vi "Read ADU Packet.vi"(8 "error in":errorcluster, 10 "isMaster (f)":bool, 11 "RTU transmission data unit in":refnum<class "RTU Data Unit.lvclass">) -> (0 "error out":errorcluster, 1 "modbus data unit":refnum<class "Modbus Data Unit.lvclass">, 3 "RTU transmission data unit out":refnum<class "RTU Data Unit.lvclass">, 5 "PDU Valid?":bool)   [LabVIEW 2021, in "RTU Data Unit.lvclass"]
doc: "This uses the protocol layer to read a modbus packet off of the bus, wrapped in the RTU transmission data unit."
uses:
  RTU Data Unit.lvclass
  D:/my_projects/projects/Algorithms/Labview/21/Modbus_v121c/Transmission Data Unit/Transmission Data Unit.lvclass
  D:/my_projects/projects/Algorithms/Labview/21/Modbus_v121c/Transmission Data Unit/Serial Interface/Serial Data Unit.lvclass
  Modbus Data Unit/Modbus Data Unit.lvclass
  Network Interface/Serial Interface/Serial Interface.lvclass
  D:/my_projects/projects/Algorithms/Labview/21/Modbus_v121c/Network Interface/Network Interface.lvclass
  Transmission Data Unit.lvclass/Transmission Data Unit.ctl
  Network Interface/Serial Interface/Serial Interface.lvclass/Serial Interface.ctl
  RTU Data Unit.lvclass/RTU Data Unit.ctl
  Serial Interface/Serial Data Unit.lvclass/Serial Data Unit.ctl
  Modbus Data Unit/Modbus Data Unit.lvclass/Modbus Data Unit.ctl
  Serial Interface/Serial acquisition states.ctl
  buffer element.ctl
  <vilib>/ErrorRing/Error Ring.xnode
  Network Interface/Network Interface.lvclass
  Serial Interface/Serial Data Unit.lvclass
  Transmission Data Unit.lvclass
  Network Protocol/Serial Shared Components/Serial Shared Components.lvlib
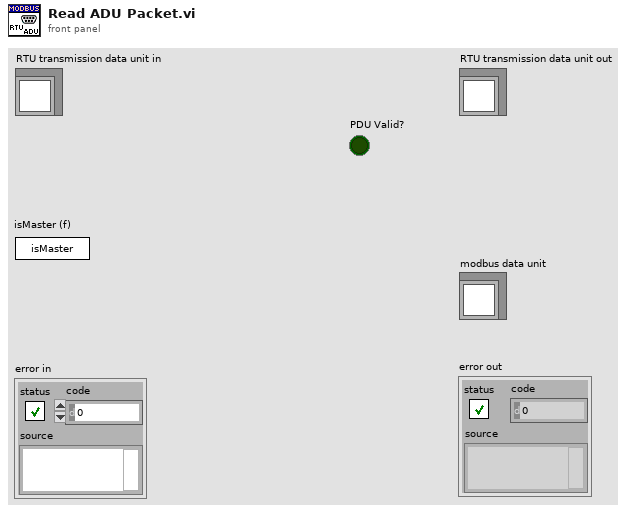
[diagram p1: front panel]
types:
  T1 = typedef "RTU Data Unit.lvclass/buffer element.ctl" = cluster{"data":u8[], "packets contained":i32}
  T2 = typedef "Serial Data Unit.lvclass/Serial acquisition states.ctl" = enum16{"Wait for frame", "Check for validity"}
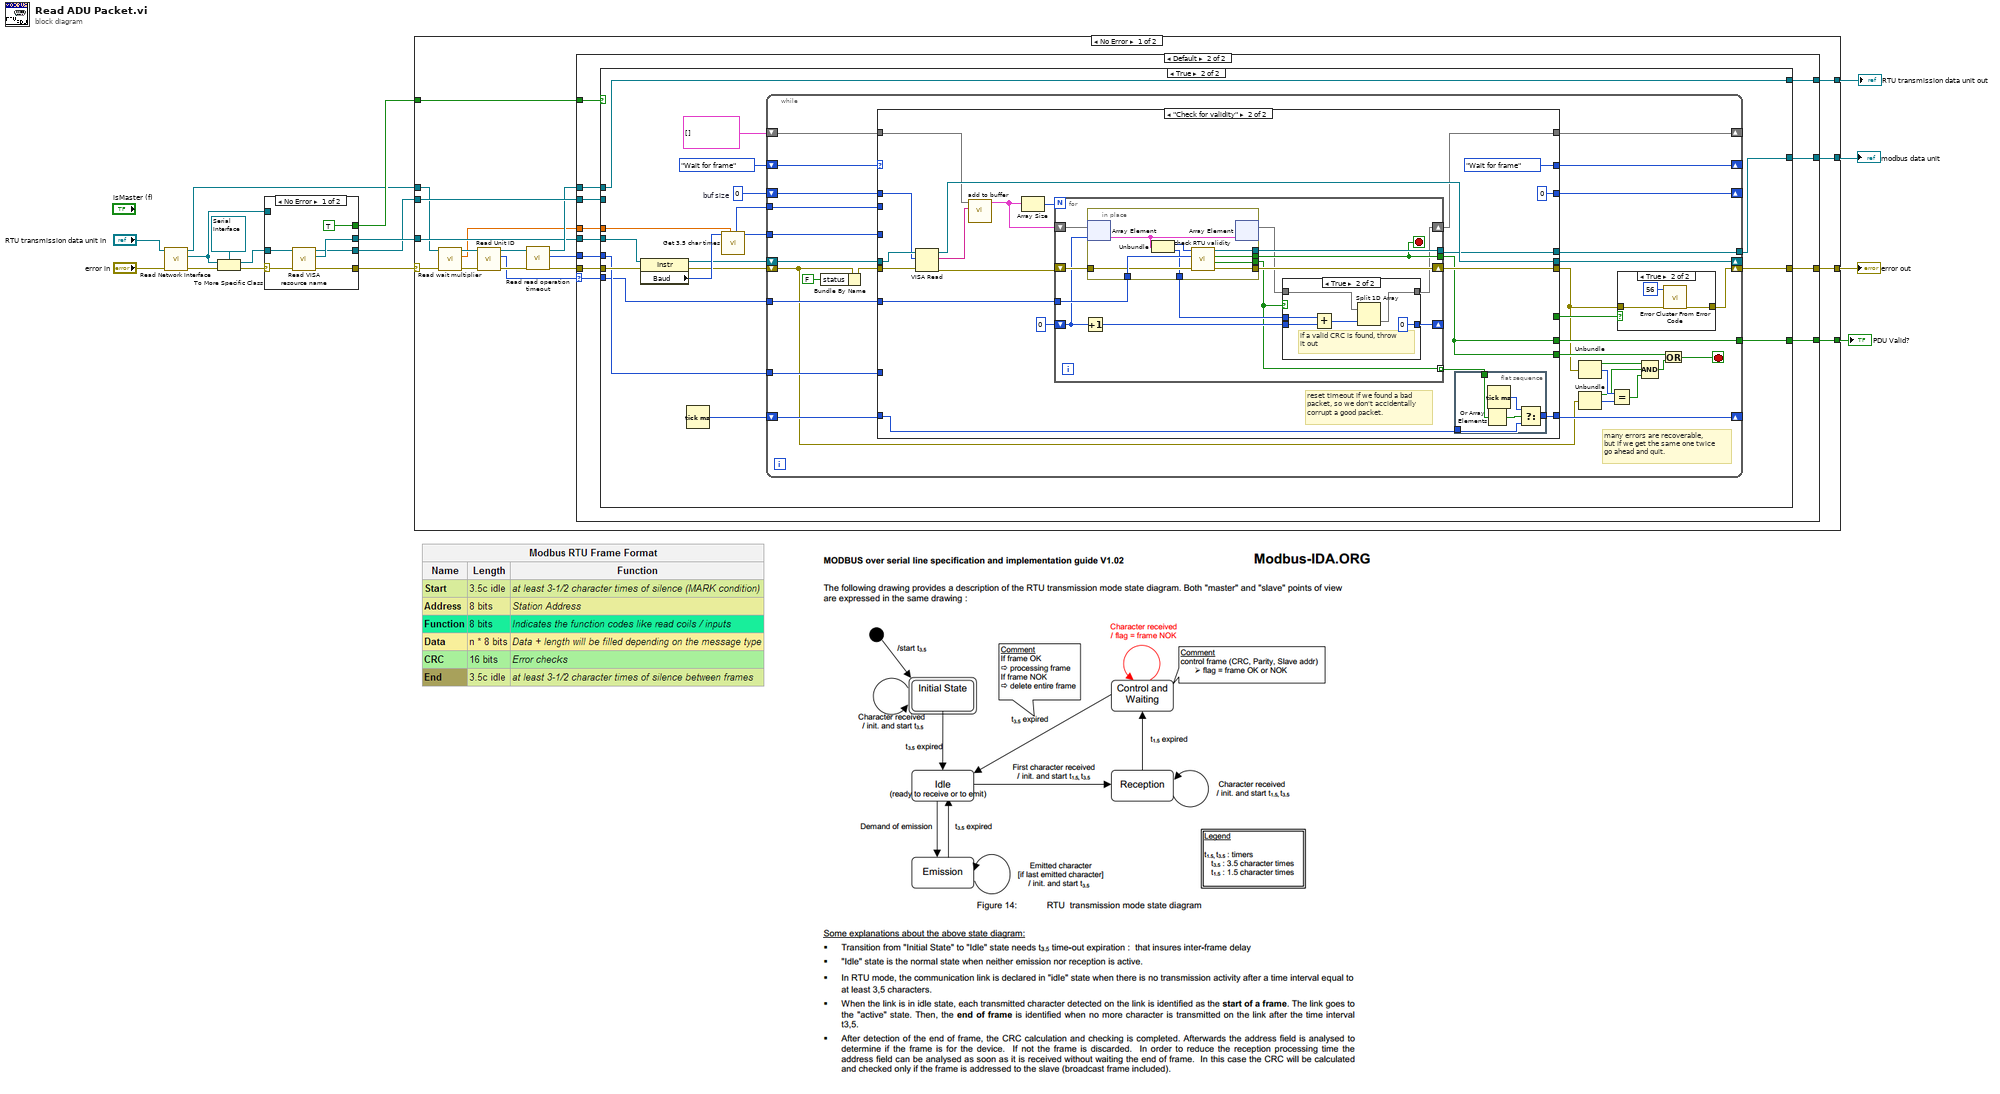
[diagram p0: block diagram]
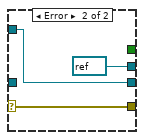
[diagram p2: hidden frame]
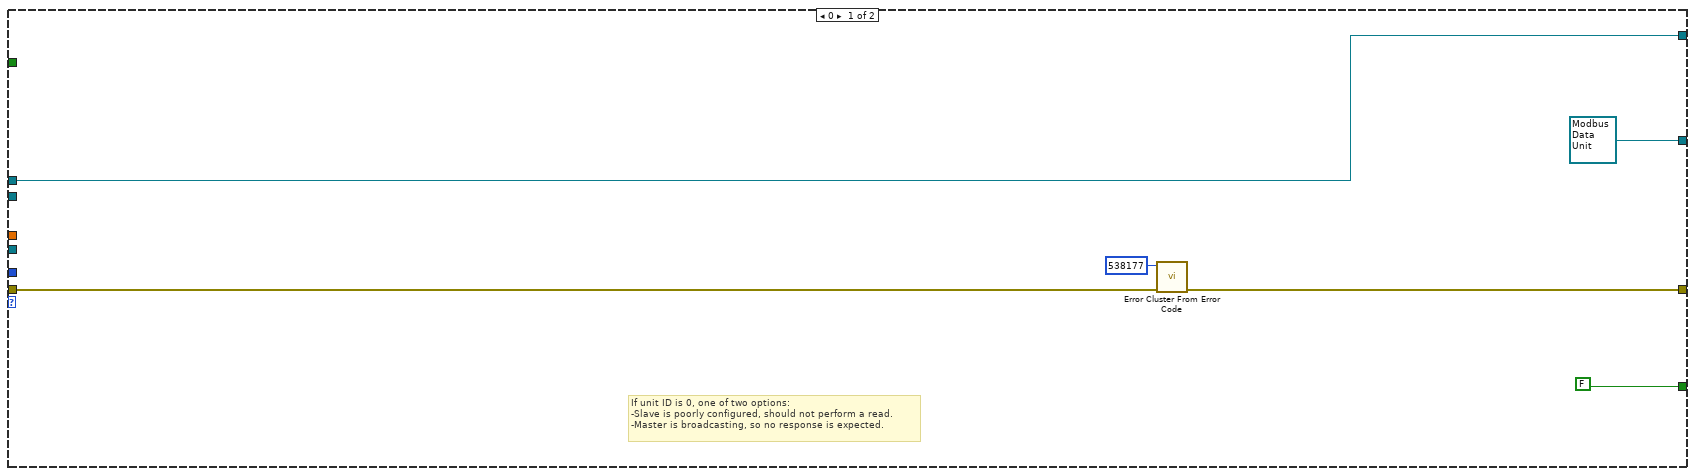
[diagram p3: hidden frame]
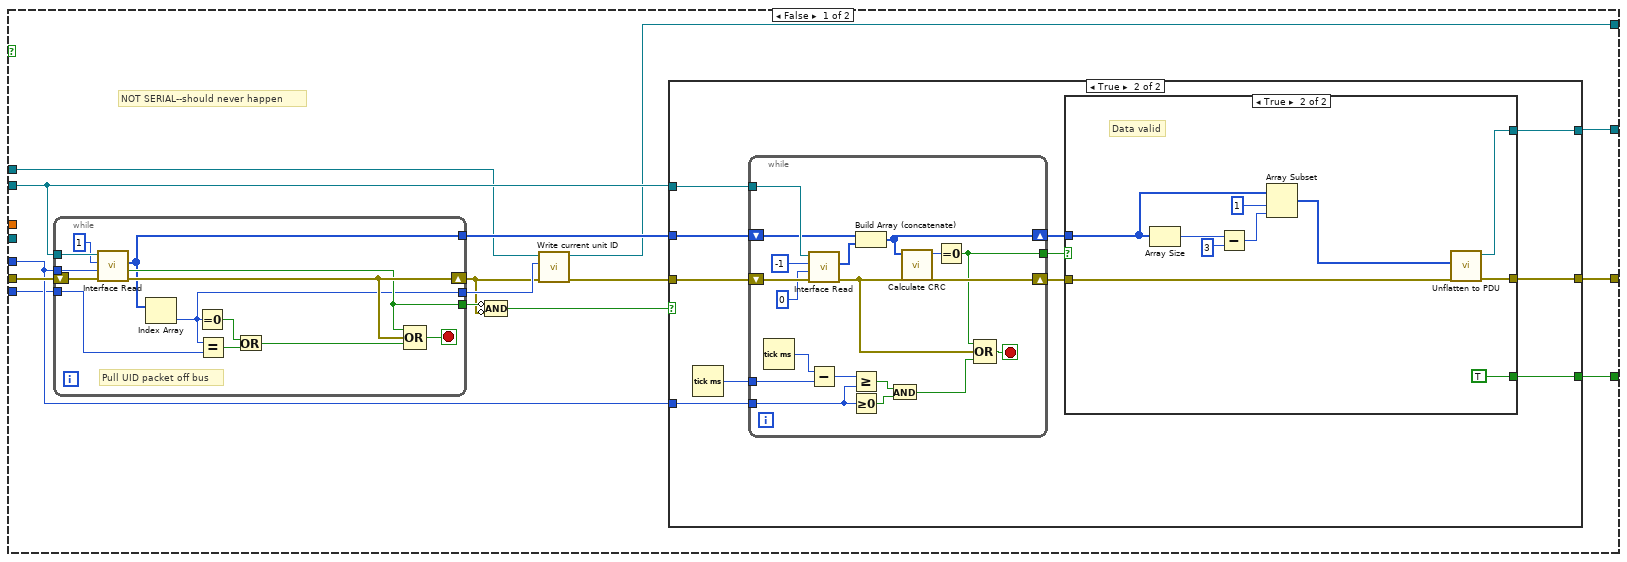
[diagram p4: hidden frame]
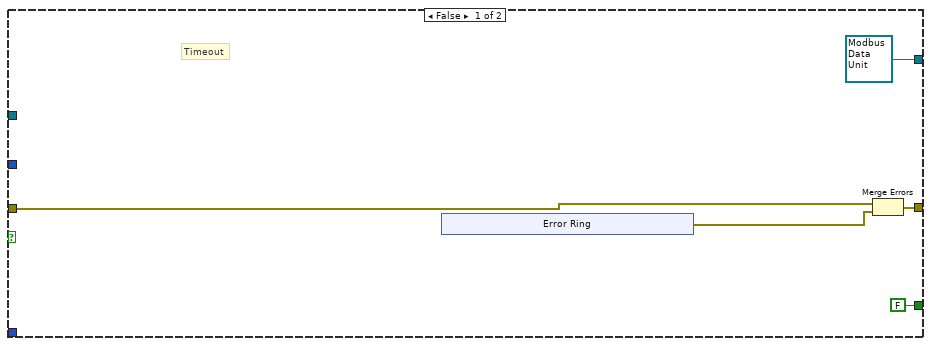
[diagram p5: hidden frame]
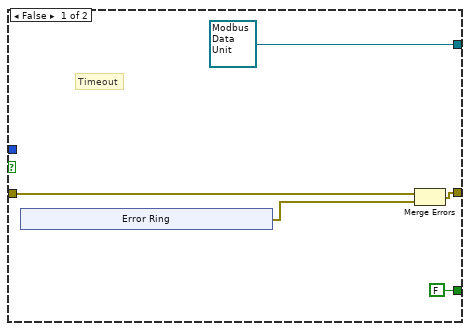
[diagram p6: hidden frame]
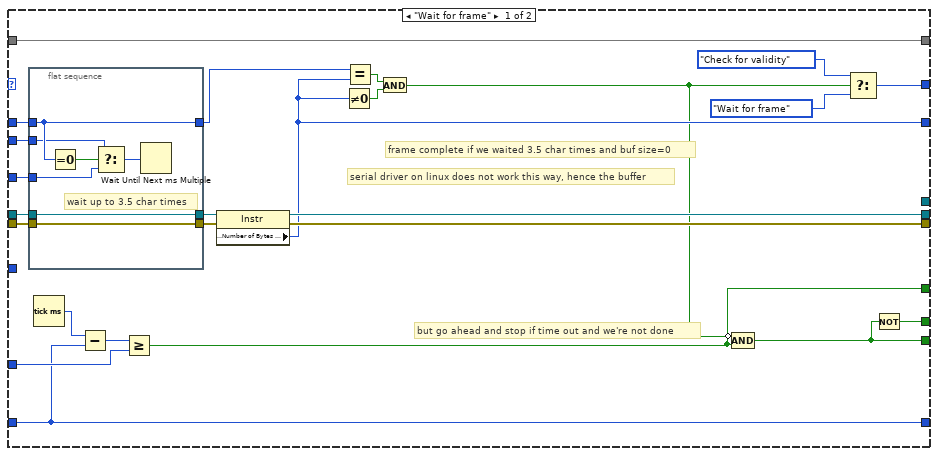
[diagram p8: hidden frame]
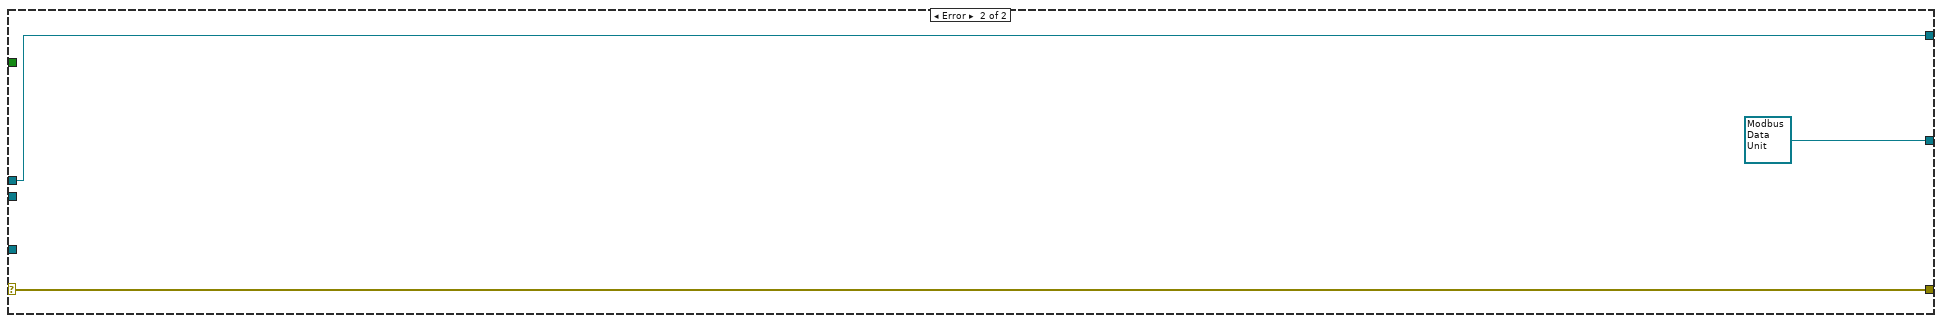
[diagram p10: hidden frame]
diagram:
  n1 = call "Read Network Interface.vi"("error in (no error)"="error in", "Transmission Data Unit in"="RTU transmission data unit in") -> ("error out"=w5:errorcluster, "Network Interface"=w4:refnum<class "Network Interface.lvclass">, "Transmission Data Unit out"=w3:refnum<class "RTU Data Unit.lvclass">)  [unwired: 7 in]
  n2 = To More Specific Class(target class=refnum<class "Serial Interface.lvclass"> refnum ("Serial Interface"), reference=w4, error in=w5) -> (specific class reference=w15:refnum<class "Serial Interface.lvclass">, error out=w16:errorcluster)
  n3 = case shown="No Error" w16 {
    selector: w16 -> [w21 w25]
    tunnel: [TRUE _] -> w13
    tunnel: [w19 refnum<visa-resource-name> refnum ("VISA resource name")] -> w14
    tunnel: w15 -> [w20 _]
    tunnel: [w18 w24] -> w1
    tunnel: [w17 w25] -> w2
    tunnel: w4 -> [_ w24]
    frame No Error {
      n4 = call "Read VISA resource name.vi"("error in (no error)"=w21, "Serial Master in"=w20) -> ("error out"=w17:errorcluster, "VISA resource name"=w19:refnum<visa-resource-name>, "Serial Master out"=w18:refnum<class "Serial Interface.lvclass">)  [unwired: 7 in]
    }
    frame Error {
    }
  }
  n5 = case shown="No Error" w2 {
    selector: w2 -> [w29 w288]
    tunnel: [w43 w288] -> w10
    tunnel: w3 -> [w30 w286]
    tunnel: w1 -> [w41 _]
    tunnel: [w42 refnum<class "Modbus Data Unit.lvclass"> refnum ("modbus data unit")] -> w11
    tunnel: [w40 w286] -> w12
    tunnel: [w33 _] -> w9
    tunnel: w13 -> [w32 _]
    tunnel: w14 -> [w31 _]
    frame No Error {
      n6 = call "Read wait multiplier.vi"("error in (no error)"=w29, "RTU Data Unit in"=w30) -> ("error out"=w28:errorcluster, "wait multiplier"=w26:sgl, "RTU Data Unit out"=w27:refnum<class "RTU Data Unit.lvclass">)  [unwired: 7 in]
      n7 = call "Read Unit ID.vi"("error in"=w28, "transmission data unit in"=w27) -> ("error out"=w37:errorcluster, "unit ID"=w35:u8, "transmission data unit out"=w36:refnum<class "RTU Data Unit.lvclass">)  [unwired: 7 in]
      n8 = call "Read read operation timeout.vi"("error in (no error)"=w37, "transmission data unit in"=w36) -> ("error out"=w38:errorcluster, "read operation timeout"=w34:i32, "transmission data unit out"=w39:refnum<class "RTU Data Unit.lvclass">)  [unwired: 7 in]
      n9 = case shown="Default" w35 {
        selector: w35 -> [_ w56]
        tunnel: w38 -> [w49 w61]
        tunnel: [w45 w60] -> w43
        tunnel: [refnum<class "Modbus Data Unit.lvclass"> refnum ("modbus data unit out") w59] -> w42
        tunnel: w41 -> [_ w58]
        tunnel: w34 -> [_ w57]
        tunnel: w39 -> [w48 w54]
        tunnel: [w48 w55] -> w40
        tunnel: [FALSE w53] -> w33
        tunnel: w32 -> [_ w52]
        tunnel: w31 -> [_ w51]
        tunnel: w26 -> [_ w50]
        frame 0 {
          # "If unit ID is 0, one of two options:\n-Slave is poorly configured, should not perform a read.\n-Master is broadcasting, so no response is expected."
          n10 = call <vilib>:"Error Cluster From Error Code.vi"("error in (no error)"=w49, "error code (0)"=538177) -> ("error out"=w45:errorcluster)  [unwired: 7 in]
        }
        frame Default {
          n11 = case shown="True" w52 {
            tunnel: w61 -> [w76 w162]
            tunnel: [w73 w159] -> w60
            tunnel: [w72 w150] -> w59
            tunnel: w58 -> [w71 _]
            tunnel: w57 -> [w69 w154]
            tunnel: w56 -> [w68 w151]
            tunnel: [w67 w164] -> w55
            tunnel: w54 -> [w65 w164]
            tunnel: [w62 w152] -> w53
            tunnel: w51 -> [_ w161]
            tunnel: w50 -> [_ w147]
            frame False {
              # "NOT SERIAL--should never happen"
              n12 = while {
                shift-right: [w143] -> w63
                shift-left: w76 -> [w146]
                tunnel: w69 -> [w141]
                tunnel: w68 -> [w137]
                tunnel: [w136] -> w75
                tunnel: [w135] -> w70
                tunnel: w71 -> [w145]
                tunnel: [w134] -> w64
                stop <- w144 stop-if-true
                # "Pull UID packet off bus"
                n13 = call-dynamic "Interface Read.vi"("error in"=w146, "timeout"=w141, "bytes to read"=1, "interface in"=w145) -> ("error out"=w143:errorcluster, "timed out?"=w136:bool, "data"=w135:u8[])  [unwired: 4 in, 1 out]
                n14 = Index Array(array=w135) -> (element=w134:u8)  [unwired: 1 in]
                n15 = Equal To 0?(x=w134) -> (x = 0?=w138:bool)
                n16 = Equal?(x=w134, y=w137) -> (x = y?=w140:bool)
                n17 = Or(x=w138, y=w140) -> (x .or. y?=w139:bool)
                n18 = Compound Arithmetic op=OR(w136, w143, w139) -> (w144:bool)
              }
              n19 = Compound Arithmetic op=AND(invert w75, invert w63) -> (w74:bool)
              n20 = call "Write current unit ID.vi"("error in"=w63, "request unit ID"=w64, "Serial Data Unit in"=w65) -> ("error out"=w66:errorcluster, "Serial Data Unit out"=w67:refnum<class "RTU Data Unit.lvclass">)  [unwired: 7 in]
              n21 = case shown="True" w74 {
                tunnel: w66 -> [w79 w96]
                tunnel: [w80 w88] -> w73
                tunnel: [refnum<class "Modbus Data Unit.lvclass"> refnum ("modbus data unit out") w89] -> w72
                tunnel: w71 -> [_ w92]
                tunnel: w70 -> [_ w93]
                tunnel: w69 -> [_ w94]
                tunnel: [FALSE w86] -> w62
                frame False {
                  # "Timeout"
                  n22 = xnode "Error Ring"() -> ("error out"=w81:errorcluster)
                  n23 = Merge Errors(w79, w81) -> (w80:errorcluster)
                }
                frame True {
                  n24 = Tick Count (ms)() -> (millisecond timer value=w95:u32)
                  n25 = while {
                    shift-right: [w119] -> w90
                    shift-left: w96 -> [w125]
                    tunnel: w95 -> [w133]
                    tunnel: w94 -> [w130]
                    shift-right: [w117] -> w87
                    shift-left: w93 -> [w121]
                    tunnel: w92 -> [w124]
                    tunnel: [w116] -> w91
                    stop <- w127 stop-if-true
                    n26 = Tick Count (ms)() -> (millisecond timer value=w132:u32)
                    n27 = call-dynamic "Interface Read.vi"("error in"=w125, "timeout"=0, "bytes to read"=-1, "interface in"=w124) -> ("error out"=w119:errorcluster, "data"=w120:u8[])  [unwired: 4 in, 2 out]
                    n28 = Subtract(x=w132, y=w133) -> (x-y=w131:u32)
                    n29 = Greater Or Equal?(x=w131, y=w130) -> (x >= y?=w128:bool)
                    n30 = Greater Or Equal To 0?(x=w130) -> (x >= 0?=w129:bool)
                    n31 = Build Array (concatenate)(w121, w120) -> (w117:u8[])
                    n32 = And(x=w128, y=w129) -> (x .and. y?=w126:bool)
                    n33 = call "Calculate CRC.vi"("data"=w117) -> ("CRC-16"=w118:u16)  [unwired: 10 in]
                    n34 = Equal To 0?(x=w118) -> (x = 0?=w116:bool)
                    n35 = Compound Arithmetic op=OR(w116, w119, w126) -> (w127:bool)
                  }
                  n36 = case shown="True" w91 {
                    tunnel: w90 -> [w99 w113]
                    tunnel: [refnum<class "Modbus Data Unit.lvclass"> refnum ("modbus data unit") w114] -> w89
                    tunnel: [w98 w115] -> w88
                    tunnel: w87 -> [_ w107]
                    tunnel: [FALSE TRUE] -> w86
                    frame False {
                      # "Timeout"
                      n37 = xnode "Error Ring"() -> ("error out"=w100:errorcluster)
                      n38 = Merge Errors(w99, w100) -> (w98:errorcluster)
                    }
                    frame True {
                      # "Data valid"
                      n39 = Array Size(array=w107) -> (size(s)=w111:i32)
                      n40 = Subtract(x=w111, y=3) -> (x-y=w109:i32)
                      n41 = Array Subset(array=w107, index=1, length=w109) -> (w108:u8[])
                      n42 = call "Unflatten to PDU.vi"("error in"=w113, "modbus data unit data"=w108) -> ("error out"=w115:errorcluster, "modbus data unit out"=w114:refnum<class "Modbus Data Unit.lvclass">)  [unwired: 8 in]
                    }
                  }
                }
              }
            }
            frame True {
              w156 = u32 0  # buf size
              n43 = property class="Instr"(reference=w161, error in=w162) -> (reference out=w158:refnum<visa-resource-name>, error out=w160:errorcluster, "Baud"=w163:u32)
              n44 = Tick Count (ms)() -> (millisecond timer value=w155:u32)
              n45 = call "Get 3.5 char times.vi"("wait multiplier"=w147, "baud rate"=w163) -> ("wait time (ms)"=w153:u32, "initial wait (ms)"=w149:u32)  [unwired: 8 in]
              n46 = while {
                shift-right: [w181] -> w159
                shift-left: w160 -> [w171]
                shift-right: [w187] -> _
                shift-left: w158 -> [w193]
                shift-right: [w186] -> _
                shift-left: Serial_acquisition_states."Wait for frame" ("Serial Acquisition States") -> [w194]
                shift-right: [w188] -> _
                shift-left: w156 -> [w190]
                tunnel: w154 -> [w191]
                tunnel: w153 -> [w189]
                tunnel: [w185] -> w152
                tunnel: w151 -> [w184]
                tunnel: [w183] -> w150
                tunnel: w149 -> [w180]
                shift-right: [w178] -> _
                shift-left: T1[] [] -> [w179]
                shift-right: [w177] -> _
                shift-left: w155 -> [w192]
                stop <- w174 stop-if-true
                # "many errors are recoverable,\nbut if we get the same one twice\ngo ahead and quit."
                n47 = Bundle By Name(cluster=w171, "status"=FALSE) -> (w176:errorcluster)
                n48 = case shown="\"Check for validity\"" w194 {
                  tunnel: w193 -> [w219 w249]
                  tunnel: w176 -> [w218 w250]
                  tunnel: w192 -> [w199 w232]
                  tunnel: w191 -> [w221 _]
                  tunnel: w190 -> [w216 w248]
                  tunnel: w189 -> [w215 _]
                  tunnel: [w206 u32 0 ("Bytes at Port")] -> w188
                  tunnel: [w203 w233] -> w173
                  tunnel: [w211 w243] -> w172
                  tunnel: [w210 w242] -> w187
                  tunnel: [w207 Serial_acquisition_states."Wait for frame" ("Serial Acquisition States")] -> w186
                  tunnel: [w204 w233] -> w185
                  tunnel: w184 -> [_ w246]
                  tunnel: [_ w240] -> w183
                  tunnel: [w202 _] -> w182
                  tunnel: w180 -> [w201 _]
                  tunnel: w179 -> [w200 w239]
                  tunnel: [w200 w235] -> w178
                  tunnel: [w199 w234] -> w177
                  frame "Wait for frame" {
                    # "serial driver on linux does not work this way, hence the buffer"
                    # "but go ahead and stop if time out and we're not done"
                    # "frame complete if we waited 3.5 char times and buf size=0"
                    n49 = flat-sequence {
                      tunnel: [w230] -> w220
                      tunnel: w219 -> [w230]
                      tunnel: w218 -> [w229]
                      tunnel: [w229] -> w217
                      tunnel: w216 -> [w228]
                      tunnel: [w228] -> w212
                      tunnel: w215 -> [w226]
                      tunnel: w201 -> [w224]
                      frame #0 {
                        # "wait up to 3.5 char times"
                        n50 = Equal To 0?(x=w228) -> (x = 0?=w227:bool)
                        n51 = Select(t=w224, s=w227, f=w226) -> (s? t:f=w225:u32)
                        n52 = Wait Until Next ms Multiple(millisecond multiple=w225) -> ()  [unwired: 1 out]
                      }
                    }
                    n53 = Tick Count (ms)() -> (millisecond timer value=w223:u32)
                    n54 = Subtract(x=w223, y=w199) -> (x-y=w222:u32)
                    n55 = Greater Or Equal?(x=w222, y=w221) -> (x >= y?=w202:bool)
                    n56 = property class="Instr"(reference=w220, error in=w217) -> (reference out=w210:refnum<visa-resource-name>, error out=w211:errorcluster, "Serial Settings:Number of Bytes at Serial Port"=w206:u32)
                    n57 = Not Equal To 0?(x=w206) -> (x != 0?=w214:bool)
                    n58 = Equal?(x=w212, y=w206) -> (x = y?=w213:bool)
                    n59 = And(x=w213, y=w214) -> (x .and. y?=w205:bool)
                    n60 = Compound Arithmetic op=AND(invert w205, w202) -> (w203:bool)
                    n61 = Select(t=Serial_acquisition_states."Check for validity" ("Serial Acquisition States"), s=w205, f=Serial_acquisition_states."Wait for frame" ("Serial Acquisition States")) -> (s? t:f=w207:T2)
                    n62 = Not(x=w203) -> (.not. x?=w204:bool)
                  }
                  frame "Check for validity" {
                    # "reset timeout if we found a bad\npacket, so we don't accidentally\ncorrupt a good packet."
                    n63 = VISA Read(VISA resource name=w249, byte count=w248, error in (no error)=w250) -> (VISA resource name out=w242:refnum<visa-resource-name>, read buffer=w247:string, error out=w245:errorcluster)  [unwired: 1 out]
                    n64 = call "add to buffer.vi"("read data"=w247, "buffer in"=w239) -> ("buffer out"=w236:T1[])  [unwired: 9 in]
                    n65 = Array Size(array=w236) -> (size(s)=w237:i32)
                    n66 = for {
                      N: w237 -> [_]
                      tunnel: w246 -> [w263]
                      tunnel: [w266] -> w240
                      shift-right: [w267] -> w243
                      shift-left: w245 -> [w268]
                      shift-right: [w258] -> _
                      shift-left: 0 -> [w262]
                      shift-right: [w259] -> w235
                      shift-left: w236 -> [w264]
                      tunnel: [w265] -> w233
                      tunnel: [w256] -> w231 mode=indexing
                      stop <- w265 stop-if-true
                      n67 = Increment(x=w262) -> (x+1=w261:i32)
                      n68 = in-place {
                        in-place-border: w263 -> [w285]
                        in-place-border: w268 -> [w284]
                        in-place-border: [w283] -> w267
                        in-place-border: [w282] -> w266
                        in-place-border: [w281] -> w265
                        in-place-border: [w280] -> w256
                        in-place-border: [w277] -> w257
                        n69 = in-place-array #1(w264, w262) -> (w279:T1)
                        n70 = Unbundle(w279) -> ("data"=w278:u8[], "packets contained"=w277:i32)
                        n71 = call "check RTU validity.vi"("error in (no error)"=w284, "unit ID"=w285, "unsigned byte array"=w278) -> ("error out"=w283:errorcluster, "valid packet"=w280:bool, "valid PDU"=w281:bool, "Modbus Data Unit out"=w282:refnum<class "Modbus Data Unit.lvclass">)  [unwired: 5 in]
                        n72 = in-place-array #1(w279) -> (w260:T1[])  [unwired: 1 out]
                      }
                      n73 = case shown="True" w256 {
                        tunnel: w260 -> [w270 w276]
                        tunnel: w261 -> [w269 w275]
                        tunnel: [w270 w273] -> w259
                        tunnel: [w269 0] -> w258
                        tunnel: w257 -> [_ w271]
                        frame False {
                        }
                        frame True {
                          # "if a valid CRC is found, throw\nit out"
                          n74 = Add(x=w271, y=w275) -> (x+y=w272:i32)
                          n75 = Split 1D Array(array=w276, index=w272) -> (second subarray=w273:T1[])  [unwired: 1 out]
                        }
                      }
                    }
                    n76 = flat-sequence {
                      tunnel: [w255] -> w234
                      tunnel: w232 -> [w254]
                      tunnel: w231 -> [w252]
                      frame #0 {
                        n77 = Or Array Elements(Boolean array=w252) -> (logical OR=w253:bool)
                        n78 = Tick Count (ms)() -> (millisecond timer value=w251:u32)
                        n79 = Select(t=w251, s=w253, f=w254) -> (s? t:f=w255:u32)
                      }
                    }
                  }
                }
                n80 = Unbundle(w172) -> ("status"=w168:bool, "code"=w169:i32)  [unwired: 1 out]
                n81 = Unbundle(w171) -> ("status"=w167:bool, "code"=w170:i32)  [unwired: 1 out]
                n82 = Equal?(x=w169, y=w170) -> (x = y?=w165:bool)
                n83 = case shown="True" w182 {
                  tunnel: w172 -> [w195 w198]
                  tunnel: [w195 w197] -> w181
                  frame False {
                  }
                  frame True {
                    n84 = call <vilib>:"Error Cluster From Error Code.vi"("error in (no error)"=w198, "error code (0)"=56) -> ("error out"=w197:errorcluster)  [unwired: 7 in]
                  }
                }
                n85 = Compound Arithmetic op=AND(w168, w167, w165) -> (w166:bool)
                n86 = Or(x=w173, y=w166) -> (x .or. y?=w174:bool)
              }
            }
          }
        }
      }
    }
    frame Error {
    }
  }
  "RTU transmission data unit out" <- w12
  "modbus data unit" <- w11
  "error out" <- w10
  "PDU Valid?" <- w9
